vi "Start DAQ.vi"(8 "error in (no error)":errorcluster, 11 "Cfg Grandmaster in":refnum<class "Cfg Grandmaster.lvclass">) -> (0 "error out":errorcluster, 3 "Cfg Grandmaster out":refnum<class "Cfg Grandmaster.lvclass">)   [LabVIEW 2012, in "Configuration Grandmaster.lvlib" / "Cfg Grandmaster.lvclass"]
uses:
  Cfg Grandmaster.lvclass
  Cfg Grandmaster.lvclass/Cfg Grandmaster.ctl
  Common/Controls/DAQMan Mode.ctl
  <vilib>/ActorFramework/Actor/Actor.lvclass/Actor.ctl
  <vilib>/ActorFramework/Message Enqueuer/Message Enqueuer.lvclass/Message Enqueuer.ctl
  Data Acquisition/Class Chassis Tasks/Chassis Tasks.lvclass
  <vilib>/ActorFramework/Message Enqueuer/Init from Existing Queue.vi
  <vilib>/ActorFramework/Message Enqueuer/Message Enqueuer.lvclass
  Class FP Ctrls/FP Controls.lvclass
  <vilib>/ActorFramework/Actor/Actor.lvclass
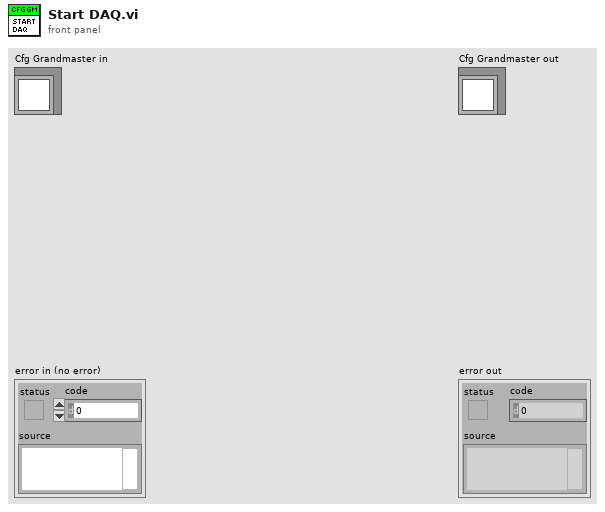
[diagram p1: front panel]
types:
  T1 = typedef "DAQMan Mode.ctl" = enum16{"Cfg", "Run", "Shutting Down"}
  T2 = typedef "ge_Cfg wChassis.ctl" = cluster{"Chassis BOM":refnum<class "Chassis BOM.lvclass">, "Chassis Cfg":refnum<class "ChassisCfg.lvclass">, "Chassis Tasks":refnum<class "Chassis Tasks.lvclass">, "HW Error":bool, "Unsvd Chgs?":bool}
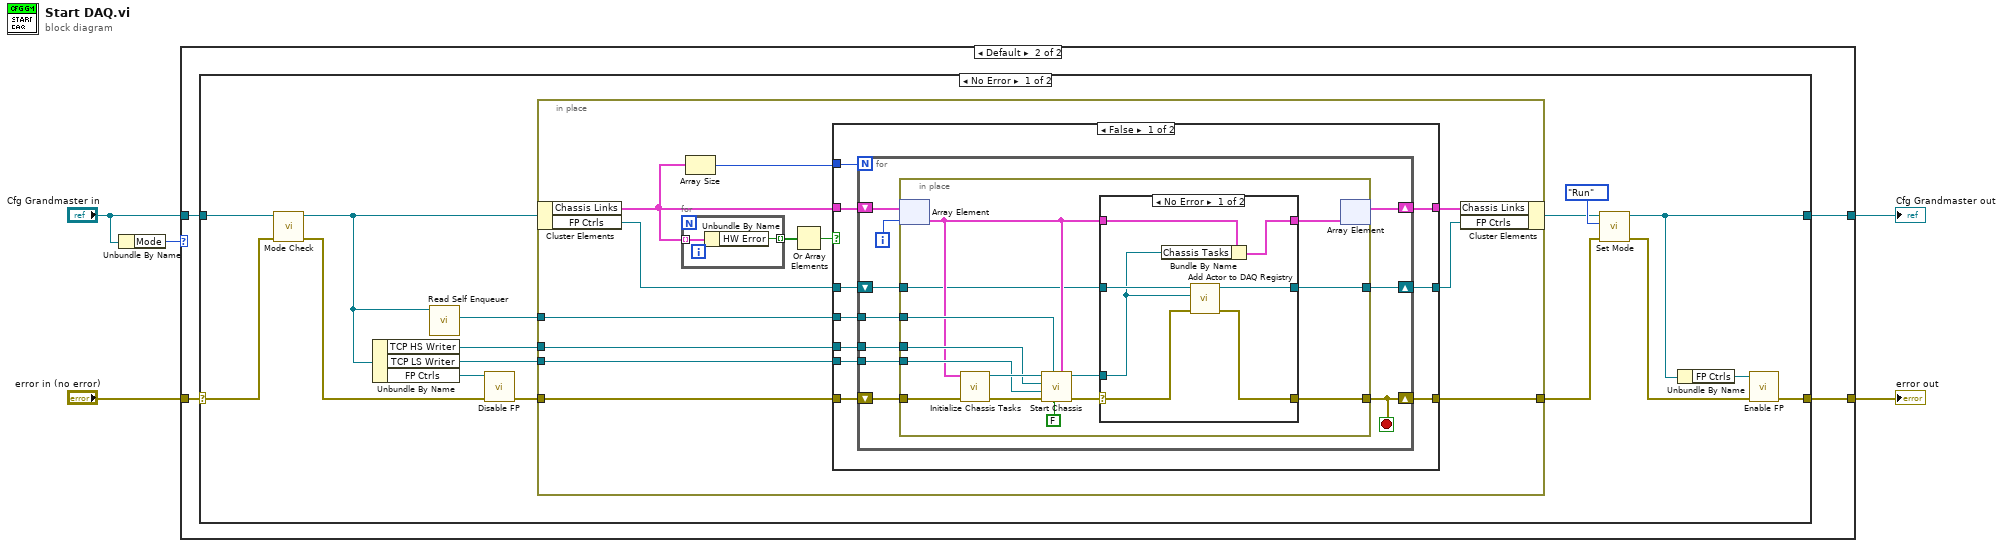
[diagram p0: block diagram]
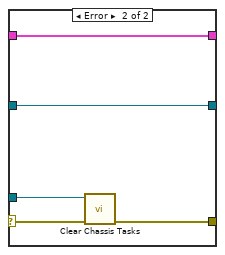
[diagram p3: hidden frame]
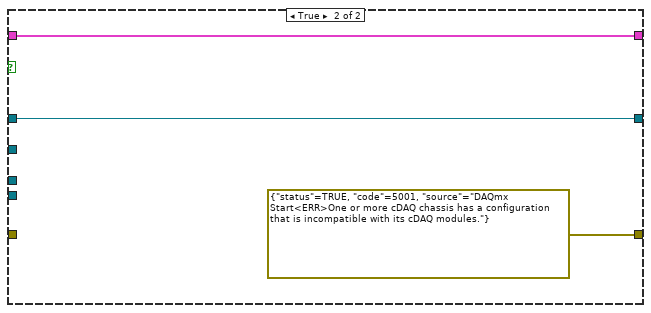
[diagram p4: hidden frame]
diagram:
  n1 = Unbundle By Name("Cfg Grandmaster in") -> ("Mode"=w1:T1)
  n2 = case shown="Default" w1 {
    tunnel: [w6 w11] -> w5
    tunnel: [w7 w10] -> w4
    tunnel: "error in (no error)" -> [w6 w9]
    tunnel: "Cfg Grandmaster in" -> [w7 w8]
    frame "Shutting Down" {
    }
    frame Default {
      n3 = case shown="No Error" w9 {
        selector: w9 -> [w19 w92]
        tunnel: [w23 w92] -> w11
        tunnel: [w13 w91] -> w10
        tunnel: w8 -> [w21 w91]
        frame No Error {
          n4 = call "Mode Check.vi"("error in (no error)"=w19, "Cfg Grandmaster in"=w21) -> ("error out"=w20:errorcluster, "Cfg Grandmaster out"=w17:refnum<class "Cfg Grandmaster.lvclass">)  [unwired: 8 in]
          n5 = Unbundle By Name(w17) -> ("TCP HS Writer"=w26:refnum<class "Message Enqueuer.lvclass">, "TCP LS Writer"=w25:refnum<class "Message Enqueuer.lvclass">, "FP Ctrls"=w24:refnum<class "FP Controls.lvclass">)
          n6 = call <vilib>:"Read Self Enqueuer.vi"("Actor"=w17) -> ("Self Enqueuer"=w27:refnum<class "Message Enqueuer.lvclass">)  [unwired: 10 in]
          n7 = call "Disable FP.vi"("error in (no error)"=w20, "FP Controls in"=w24) -> ("error out"=w18:errorcluster)  [unwired: 8 in, 1 out]
          n8 = in-place {
            in-place-border: [w37] -> w14
            in-place-border: w18 -> [w36]
            in-place-border: w27 -> [w35]
            in-place-border: w26 -> [w34]
            in-place-border: w25 -> [w33]
            n9 = in-place-cluster #1(w17) -> ("Chassis Links"=w31:T2[], "FP Ctrls"=w29:refnum<class "FP Controls.lvclass">)
            n10 = for {
              tunnel: w31 -> [w90] mode=indexing
              tunnel: [w89] -> w38 mode=indexing
              n11 = Unbundle By Name(w90) -> ("HW Error"=w89:bool)
            }
            n12 = Array Size(array=w31) -> (size(s)=w30:i32)
            n13 = Or Array Elements(Boolean array=w38) -> (logical OR=w39:bool)
            n14 = case shown="False" w39 {
              tunnel: w36 -> [w48 _]
              tunnel: [w44 errorcluster {"status"=TRUE, "code"=5001, "source"="DAQmx Start<ERR>One or more cDAQ chassis has a configuration that is incompatible with its cDAQ modules."} ("error IO")] -> w37
              tunnel: w31 -> [w49 w87]
              tunnel: [w43 w87] -> w32
              tunnel: w35 -> [w47 _]
              tunnel: w34 -> [w46 _]
              tunnel: w33 -> [w45 _]
              tunnel: w30 -> [w42 _]
              tunnel: w29 -> [w41 w86]
              tunnel: [w40 w86] -> w28
              frame False {
                n15 = for {
                  N: w42 -> [_]
                  shift-right: [w52] -> w44
                  shift-left: w48 -> [w59]
                  tunnel: w47 -> [w58]
                  tunnel: w46 -> [w57]
                  tunnel: w45 -> [w56]
                  shift-right: [w54] -> w43
                  shift-left: w49 -> [w55]
                  shift-right: [w50] -> w40
                  shift-left: w41 -> [w51]
                  i -> [w53]
                  stop <- w52 stop-if-true
                  n16 = in-place {
                    in-place-border: [w72] -> w52
                    in-place-border: w59 -> [w71]
                    in-place-border: w58 -> [w69]
                    in-place-border: w57 -> [w68]
                    in-place-border: w56 -> [w67]
                    in-place-border: w51 -> [w63]
                    in-place-border: [w64] -> w50
                    n17 = in-place-array #2(w55, w53) -> (w66:T2)
                    n18 = call "Initialize Chassis Tasks.vi"("error in"=w71, "Cfg wChassis"=w66) -> ("error out"=w73:errorcluster, "Chassis Tasks out"=w70:refnum<class "Chassis Tasks.lvclass">)  [unwired: 8 in]
                    n19 = call-dynamic "Start Chassis.vi"("Cfg wChassis"=w66, "Show FP?"=FALSE, "Actor-to-Caller Enqueuer"=w69, "error in (no error)"=w73, "TCP LS Writer"=w67, "TCP HS Writer"=w68, "Chassis Tasks in"=w70) -> ("error out"=w60:errorcluster, "Chassis Tasks out"=w62:refnum<class "Chassis Tasks.lvclass">)  [unwired: 3 in]
                    n20 = case shown="No Error" w60 {
                      selector: w60 -> [w74 w83]
                      tunnel: [w80 w81] -> w72
                      tunnel: w66 -> [w79 w85]
                      tunnel: [w78 w85] -> w65
                      tunnel: [w77 w84] -> w64
                      tunnel: w63 -> [w76 w84]
                      tunnel: w62 -> [w75 w82]
                      frame No Error {
                        n21 = Bundle By Name(cluster=w79, "Chassis Tasks"=w75) -> (w78:T2)
                        n22 = call "Add Actor to DAQ Registry.vi"("error in (no error)"=w74, "Chassis Tasks out"=w75, "FP Controls in"=w76) -> ("error out"=w80:errorcluster, "FP Controls out"=w77:refnum<class "FP Controls.lvclass">)  [unwired: 7 in]
                      }
                      frame Error {
                        n23 = call "Clear Chassis Tasks.vi"("error in (no error)"=w83, "Chassis Tasks in"=w82) -> ("error out"=w81:errorcluster)  [unwired: 8 in, 1 out]
                      }
                    }
                    n24 = in-place-array #2(w65) -> (w54:T2[])  [unwired: 1 out]
                  }
                }
              }
              frame True {
              }
            }
            n25 = in-place-cluster #1("Chassis Links"=w32, "FP Ctrls"=w28) -> (w15:refnum<class "Cfg Grandmaster.lvclass">)
          }
          n26 = call "Set Mode.vi"("error in (no error)"=w14, "Mode"=DAQMan_Mode."Run", "Cfg Grandmaster in"=w15) -> ("error out"=w12:errorcluster, "Cfg Grandmaster out"=w13:refnum<class "Cfg Grandmaster.lvclass">)  [unwired: 7 in]
          n27 = Unbundle By Name(w13) -> ("FP Ctrls"=w22:refnum<class "FP Controls.lvclass">)
          n28 = call "Enable FP.vi"("error in (no error)"=w12, "FP Controls in"=w22) -> ("error out"=w23:errorcluster)  [unwired: 8 in, 1 out]
        }
        frame Error {
        }
      }
    }
  }
  "error out" <- w5
  "Cfg Grandmaster out" <- w4
